vi "writeToXML.vi"(8 "error in (no error)":errorcluster, 10 "ClassLabel":string, 11 "TCSWeatherServerCommand in":refnum<class "TCSWeatherServerCommand.lvclass">) -> (0 "error out":errorcluster, 2 "XMLout":string, 3 "TCSWeatherServerCommand out":refnum<class "TCSWeatherServerCommand.lvclass">)   [LabVIEW 2014, in "TCSDataDefinitions.lvlib" / "TCSWeatherServerCommand.lvlib" / "TCSWeatherServerCommand.lvclass"]
uses:
  TCSWeatherServerCommand.lvclass
  TCSCommand/TCSCommand/TCSCommand.lvclass
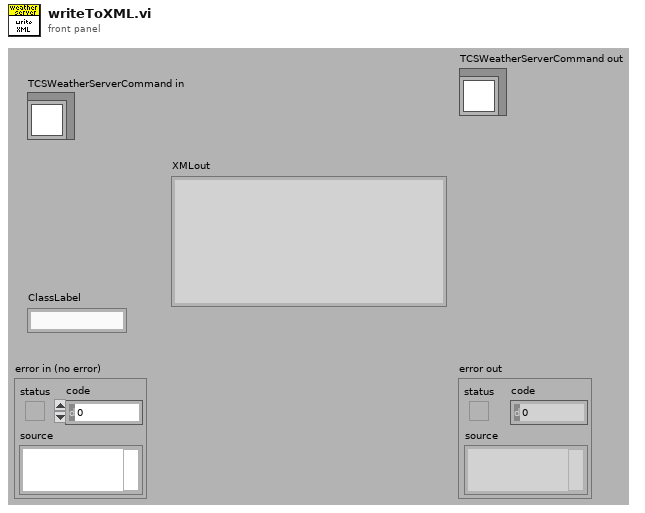
[diagram p1: front panel]
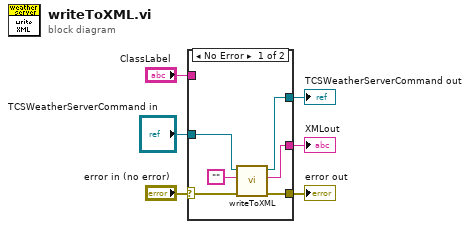
[diagram p0: block diagram]
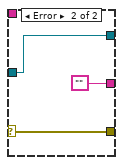
[diagram p2: hidden frame]
diagram:
  n1 = case shown="No Error" "error in (no error)" {
    selector: "error in (no error)" -> [w9 w15]
    tunnel: [w8 w15] -> w5
    tunnel: [w11 w14] -> w4
    tunnel: "TCSWeatherServerCommand in" -> [w12 w14]
    tunnel: [w7 ""] -> w3
    tunnel: "ClassLabel" -> [_ _]
    frame No Error {
      n2 = call-parent "writeToXML.vi"("error in (no error)"=w9, "Class Label"="", "TCSCommand in"=w12) -> ("error out"=w8:errorcluster, "XML out"=w7:string, "TCSCommand out"=w11:refnum<class "TCSWeatherServerCommand.lvclass">)  [unwired: 6 in]
    }
    frame Error {
    }
  }
  "error out" <- w5
  "TCSWeatherServerCommand out" <- w4
  "XMLout" <- w3
